vi "__TEST-Launcher.vi"(11 "CommandLine":string[](array[string])) -> (2 "test details":string, 3 "exit code":i32)   [LabVIEW 2019]
uses:
  <vilib>/addons/_JKI Toolkits/VI Tester/VI Tester API.llb/Run Tests (Path).vi
  <vilib>/addons/_JKI Toolkits/VI Tester/VI Tester API.llb/VI Tester API.lvlib
panel:
  out "error out":errorcluster
  in  "error in (no error)":errorcluster
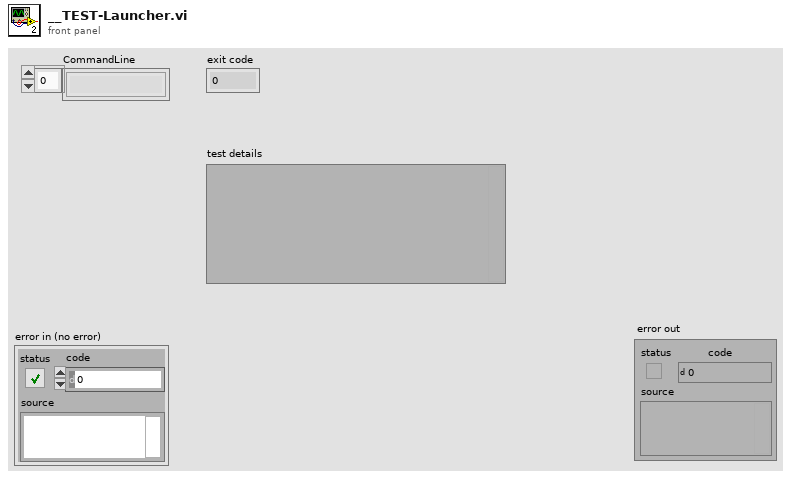
[diagram p1: front panel]
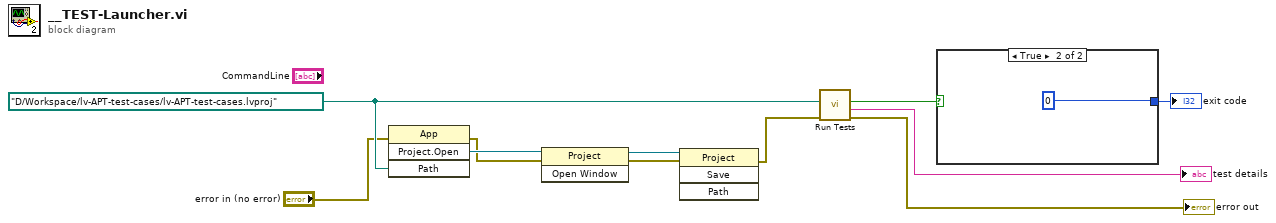
[diagram p0: block diagram]
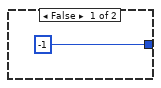
[diagram p2: hidden frame]
diagram:
  w4 = path "D:/Workspace/lv-APT-test-cases/lv-APT-test-cases.lvproj" ("Test Path")
  n1 = invoke class="App" method="Project.Open"(error in="error in (no error)", "Path"=w4) -> (error out=w5:errorcluster, "Project:Open"=w8:refnum<vi>)  [unwired: 2 in, 2 out]
  n2 = invoke class="Project" method="Open Window"(reference=w8, error in=w5) -> (reference out=w7:refnum<vi>, error out=w6:errorcluster)  [unwired: 1 in, 1 out]
  n3 = invoke class="Project" method="Save"(reference=w7, error in=w6) -> (error out=w3:errorcluster)  [unwired: 2 in, 3 out]
  n4 = call-poly <vilib>:"Run Tests.vi"("error in (no error)"=w3, "Test Path"=w4) -> ("error out"=→"error out":errorcluster, "test details"=→"test details":string, "successful?"=w10:bool)  [unwired: 7 in]
  n5 = case shown="True" w10 {
    tunnel: [-1 0] -> w9
    frame False {
    }
    frame True {
    }
  }
  "exit code" <- w9
